vi "405Pico.vi"() -> ()   [LabVIEW 2013]
panel:
  out "405":bool
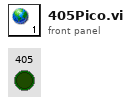
[diagram p1: front panel]
diagram:
